vi "Configure Source Limit Level.vi"(8 "error in (no error)":errorcluster, 9 "Source Limit (1.0)":dbl=1.0, 10 "Function (0: Volts)":u16(ring) items=["Volts", "Current"], 11 "VISA resource name":refnum<visa-resource-name>) -> (0 "error out":errorcluster, 3 "VISA resource name out":refnum<visa-resource-name>)   [LabVIEW 2020, in "Keithley 2450.lvlib"]
doc: "Configures the source limit on the instrument."
uses:
  Keithley 2450.lvlib
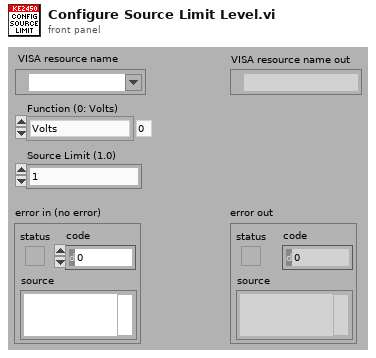
[diagram p1: front panel]
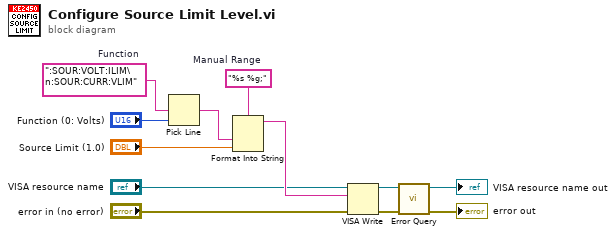
[diagram p0: block diagram]
diagram:
  w8 = ":SOUR:VOLT:ILIM\n:SOUR:CURR:VLIM"  # Function
  w9 = "%s %g;"  # Manual Range
  n1 = Pick Line(multi-line string=w8, line index="Function (0: Volts)") -> (output string=w7:string)  [unwired: 1 out]
  n2 = Format Into String(format string=w9, w7, "Source Limit (1.0)") -> (resulting string=w10:string)  [unwired: 2 in, 1 out]
  n3 = VISA Write(VISA resource name="VISA resource name", write buffer=w10, error in (no error)="error in (no error)") -> (VISA resource name out=w4:refnum<visa-resource-name>, error out=w3:errorcluster)  [unwired: 1 out]
  n4 = call "Error Query.vi"("error in (no error)"=w3, "VISA resource name"=w4) -> ("error out"=→"error out":errorcluster, "VISA resource name out"=→"VISA resource name out":refnum<visa-resource-name>)  [unwired: 8 out]
